vi "SetValue.vi"(8 "error in":errorcluster, 10 "Value":T1, 11 "Measure in":refnum<class "MeasureKind.lvclass">) -> (0 "error out":errorcluster, 3 "Measure out":refnum<class "MeasureKind.lvclass">)   [LabVIEW 2021, in "ProligentXMLGenerator.lvlib" / "MeasureKind.lvclass"]
uses:
  MeasureKind.lvclass
  MeasureKind.lvclass/MeasureKind.ctl
  Value.ctl
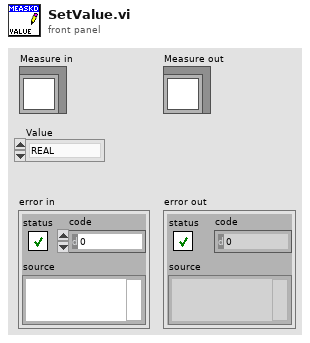
[diagram p1: front panel]
types:
  T1 = typedef "ProligentXMLGenerator.lvlib/MeasureKind.lvclass/Value.ctl" = enum16{"REAL", "BOOL", "INTEGER", "STRING", "DATETIME"}
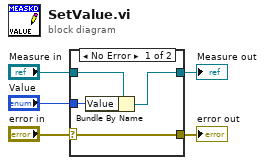
[diagram p0: block diagram]
diagram:
  n1 = case shown="No Error" "error in" {
    selector: "error in" -> [w6 w10]
    tunnel: "Measure in" -> [w9 w11]
    tunnel: [w8 w11] -> w1
    tunnel: "Value" -> [w7 _]
    tunnel: [w6 w10] -> w2
    frame No Error {
      n2 = Bundle By Name(cluster=w9, "Value"=w7) -> (w8:refnum<class "MeasureKind.lvclass">)
    }
    frame Error {
    }
  }
  "error out" <- w2
  "Measure out" <- w1
